vi "Post-Install Custom Action.vi"(10 "Variant":variant) -> (0 "error out":errorcluster)   [LabVIEW 2015]
uses:
  <vilib>/Palette API/Palette Menu/Public Type Define/Palette type.ctl
  <vilib>/Palette API/Palette Menu/Public Type Define/Item.ctl
  <vilib>/Palette API/Palette Menu/Palette Menu.lvlib
panel:
  out "error out 2":errorcluster
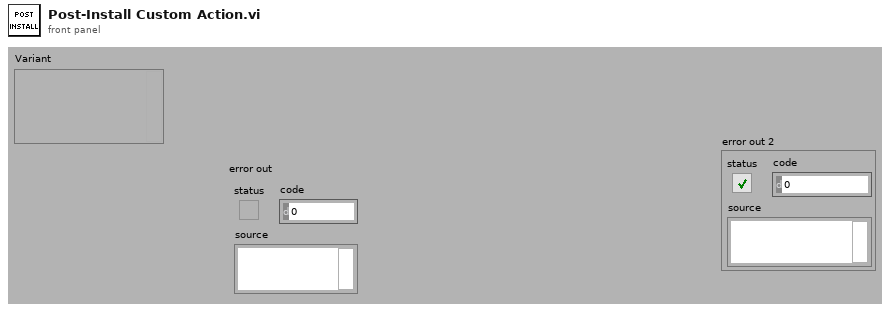
[diagram p1: front panel]
types:
  T1 = typedef "Palette Menu.lvlib/Palette type.ctl" = i32
  T2 = typedef "Palette Menu.lvlib/Palette Data.ctl" = cluster{"display name":string, "view format":T3, "palette width":i16, "items":T4, "256 color icon":picture, "B&W color icon":picture, "help information":T6, "palette description":string, "synchronize information":T7}
  T3 = typedef "Palette Menu.lvlib/View Format.ctl" = u16
  T4 = typedef "Palette Menu.lvlib/Items.ctl" = T5[]
  T5 = typedef "Palette Menu.lvlib/Item.ctl" = cluster{"item path":path, "library path (.lvlib)":path, "use default lvlib palette":bool, "short name":string, "place VI contents":bool, "hide synchronized item":bool, "reserve spot for synch item":bool, "configure when placing VI contents":bool}
  T6 = typedef "Palette Menu.lvlib/Help Info.ctl" = cluster{"help tag":string, "help file path ":path}
  T7 = typedef "Palette Menu.lvlib/Synchronize Info.ctl" = cluster{"synchronize with directory":bool, "synchronize directory path":path}
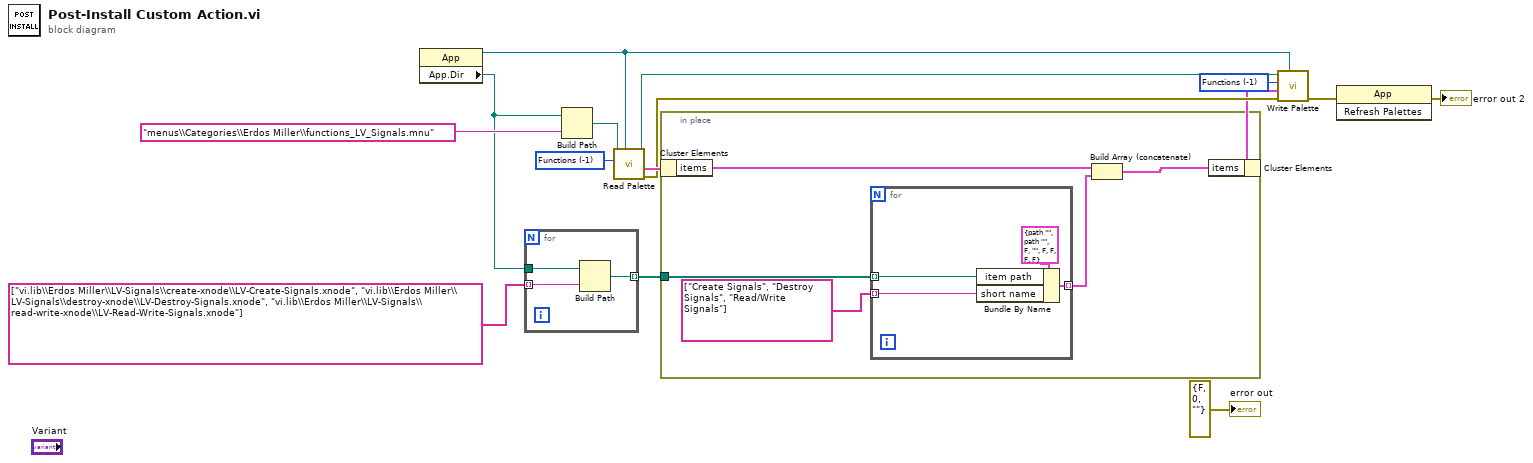
[diagram p0: block diagram]
diagram:
  w7 = T1 -1 items=["Functions"=-1, "Controls"=-2] ("palette type")
  w8 = T1 -1 items=["Functions"=-1, "Controls"=-2] ("palette type")
  n1 = property class="App"() -> (reference out=w9:refnum<vi>, "App.Dir"=w12:path)  [unwired: 2 in, 1 out]
  n2 = for {
    tunnel: string[] ["vi.lib\\Erdos Miller\\LV-Signals\\create-xnode\\LV-Create-Signals.xnode", "vi.lib\\Erdos Miller\\LV-Signals\\destroy-xnode\\LV-Destroy-Signals.xnode", "vi.lib\\Erdos Miller\\LV-Signals\\read-write-xnode\\LV-Read-Write-Signals.xnode"] -> [w17] mode=indexing
    tunnel: w12 -> [w18]
    tunnel: [w16] -> w4 mode=indexing
    n3 = Build Path(base path=w18, name or relative path=w17) -> (appended path=w16:path)
  }
  n4 = Build Path(base path=w12, name or relative path="menus\\Categories\\Erdos Miller\\functions_LV_Signals.mnu") -> (appended path=w3:path)
  n5 = call <vilib>:"Read Palette.vi"("application reference"=w9, "palette type"=w7, "palette path"=w3) -> ("error out"=w10:errorcluster, "palette data"=w13:T2, "duplicate palette path"=w11:path)  [unwired: 6 in]
  n6 = in-place {
    in-place-border: w4 -> [w23]
    n7 = in-place-cluster #1(w13) -> ("items"=w22:T4)
    n8 = for {
      tunnel: w23 -> [w26] mode=indexing
      tunnel: [w25] -> w21 mode=indexing
      tunnel: string[] ["Create Signals", "Destroy Signals", "Read/Write Signals"] -> [w24] mode=indexing
      n9 = Bundle By Name(cluster=T5 {"item path"=path "", "library path (.lvlib)"=path "", "use default lvlib palette"=FALSE, "short name"="", "place VI contents"=FALSE, "hide synchronized item"=FALSE, "reserve spot for synch item"=FALSE, "configure when placing VI contents"=FALSE} ("Items"), "item path"=w26, "short name"=w24) -> (w25:T5)
    }
    n10 = Build Array (concatenate)(w22, w21) -> (w20:T4)
    n11 = in-place-cluster #1("items"=w20) -> (w5:T2)
  }
  n12 = call <vilib>:"Write Palette.vi"("application reference"=w9, "error in (no error)"=w10, "palette data"=w5, "palette type"=w8, "palette path"=w11) -> ("error out"=w6:errorcluster)  [unwired: 6 in]
  n13 = invoke class="App" method="Refresh Palettes"(error in=w6) -> (error out=→"error out 2":errorcluster)  [unwired: 2 in, 2 out]
  "error out" <- errorcluster {"status"=FALSE, "code"=0, "source"=""} ("error out")
